vi "active_on_.vi"() -> ()   [LabVIEW 2024]
panel:
  in  "Active ON?":bool
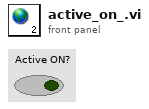
[diagram p1: front panel]
diagram:
